vi "Trio - Set Connection Parameters.vi"(9 "TrioData In":T1 {"A Axis Parameters"."VPSPEED" format="%#_4g"; "A Axis Parameters"."AXISSTATUS" format="%#_4g"; "A Axis Parameters"."FE" format="%#_4g"; "A Axis Parameters"."MPOS" format="%#_4g"; "A Axis Parameters"."NTYPE" format="%#_4g"; "A Axis Parameters"."MTYPE" format="%#_4g"; "A Axis Parameters"."RS_LIMIT" format="%#_4g"; "A Axis Parameters"."FS_LIMIT" format="%#_4g"; "A Axis Parameters"."FH_IN" format="%#_4g"; "A Axis Parameters"."DATUM_IN" format="%#_4g"; "A Axis Parameters"."REV_IN" format="%#_4g"; "A Axis Parameters"."FWD_IN" format="%#_4g"; "A Axis Parameters"."REP_DIST" format="%#_4g"; "A Axis Parameters"."SERVO" format="%#_4g"; "A Axis Parameters"."DAC" format="%#_4g"; "A Axis Parameters"."FE_LIMIT" format="%#_4g"; "A Axis Parameters"."JOGSPEED" format="%#_4g"; "A Axis Parameters"."CREEP" format="%#_4g"; "A Axis Parameters"."DECEL" format="%#_4g"; "A Axis Parameters"."ACCEL" format="%#_4g"; "A Axis Parameters"."SPEED" format="%#_4g"; "A Axis Parameters"."UNITS" format="%#_4g"; "A Axis Parameters"."VFF_GAIN" format="%#_4g"; "A Axis Parameters"."0V_GAIN" format="%#_4g"; "A Axis Parameters"."D_GAIN" format="%#_4g"; "A Axis Parameters"."I_GAIN" format="%#_4g"; "A Axis Parameters"."P_GAIN" format="%#_4g"; "A Axis Parameters"."ATYPE" format="%#_4g"; "X Axis Parameters"."VPSPEED" format="%#_4g"; "X Axis Parameters"."AXISSTATUS" format="%#_4g"; "X Axis Parameters"."FE" format="%#_4g"; "X Axis Parameters"."MPOS" format="%#_4g"; "X Axis Parameters"."NTYPE" format="%#_4g"; "X Axis Parameters"."MTYPE" format="%#_4g"; "X Axis Parameters"."RS_LIMIT" format="%#_4g"; "X Axis Parameters"."FS_LIMIT" format="%#_4g"; "X Axis Parameters"."FH_IN" format="%#_4g"; "X Axis Parameters"."DATUM_IN" format="%#_4g"; "X Axis Parameters"."REV_IN" format="%#_4g"; "X Axis Parameters"."FWD_IN" format="%#_4g"; "X Axis Parameters"."REP_DIST" format="%#_4g"; "X Axis Parameters"."SERVO" format="%#_4g"; "X Axis Parameters"."DAC" format="%#_4g"; "X Axis Parameters"."FE_LIMIT" format="%#_4g"; "X Axis Parameters"."JOGSPEED" format="%#_4g"; "X Axis Parameters"."CREEP" format="%#_4g"; "X Axis Parameters"."DECEL" format="%#_4g"; "X Axis Parameters"."ACCEL" format="%#_4g"; "X Axis Parameters"."SPEED" format="%#_4g"; "X Axis Parameters"."UNITS" format="%#_4g"; "X Axis Parameters"."VFF_GAIN" format="%#_4g"; "X Axis Parameters"."0V_GAIN" format="%#_4g"; "X Axis Parameters"."D_GAIN" format="%#_4g"; "X Axis Parameters"."I_GAIN" format="%#_4g"; "X Axis Parameters"."P_GAIN" format="%#_4g"; "X Axis Parameters"."ATYPE" format="%#_4g"}, 10 "error in (no error)":errorcluster, 11 "TrioControl Refnum in":refnum<k7>) -> (1 "TrioData Out":T1 {"A Axis Parameters"."VPSPEED" format="%#_4g"; "A Axis Parameters"."AXISSTATUS" format="%#_4g"; "A Axis Parameters"."FE" format="%#_4g"; "A Axis Parameters"."MPOS" format="%#_4g"; "A Axis Parameters"."NTYPE" format="%#_4g"; "A Axis Parameters"."MTYPE" format="%#_4g"; "A Axis Parameters"."RS_LIMIT" format="%#_4g"; "A Axis Parameters"."FS_LIMIT" format="%#_4g"; "A Axis Parameters"."FH_IN" format="%#_4g"; "A Axis Parameters"."DATUM_IN" format="%#_4g"; "A Axis Parameters"."REV_IN" format="%#_4g"; "A Axis Parameters"."FWD_IN" format="%#_4g"; "A Axis Parameters"."REP_DIST" format="%#_4g"; "A Axis Parameters"."SERVO" format="%#_4g"; "A Axis Parameters"."DAC" format="%#_4g"; "A Axis Parameters"."FE_LIMIT" format="%#_4g"; "A Axis Parameters"."JOGSPEED" format="%#_4g"; "A Axis Parameters"."CREEP" format="%#_4g"; "A Axis Parameters"."DECEL" format="%#_4g"; "A Axis Parameters"."ACCEL" format="%#_4g"; "A Axis Parameters"."SPEED" format="%#_4g"; "A Axis Parameters"."UNITS" format="%#_4g"; "A Axis Parameters"."VFF_GAIN" format="%#_4g"; "A Axis Parameters"."0V_GAIN" format="%#_4g"; "A Axis Parameters"."D_GAIN" format="%#_4g"; "A Axis Parameters"."I_GAIN" format="%#_4g"; "A Axis Parameters"."P_GAIN" format="%#_4g"; "A Axis Parameters"."ATYPE" format="%#_4g"; "X Axis Parameters"."VPSPEED" format="%#_4g"; "X Axis Parameters"."AXISSTATUS" format="%#_4g"; "X Axis Parameters"."FE" format="%#_4g"; "X Axis Parameters"."MPOS" format="%#_4g"; "X Axis Parameters"."NTYPE" format="%#_4g"; "X Axis Parameters"."MTYPE" format="%#_4g"; "X Axis Parameters"."RS_LIMIT" format="%#_4g"; "X Axis Parameters"."FS_LIMIT" format="%#_4g"; "X Axis Parameters"."FH_IN" format="%#_4g"; "X Axis Parameters"."DATUM_IN" format="%#_4g"; "X Axis Parameters"."REV_IN" format="%#_4g"; "X Axis Parameters"."FWD_IN" format="%#_4g"; "X Axis Parameters"."REP_DIST" format="%#_4g"; "X Axis Parameters"."SERVO" format="%#_4g"; "X Axis Parameters"."DAC" format="%#_4g"; "X Axis Parameters"."FE_LIMIT" format="%#_4g"; "X Axis Parameters"."JOGSPEED" format="%#_4g"; "X Axis Parameters"."CREEP" format="%#_4g"; "X Axis Parameters"."DECEL" format="%#_4g"; "X Axis Parameters"."ACCEL" format="%#_4g"; "X Axis Parameters"."SPEED" format="%#_4g"; "X Axis Parameters"."UNITS" format="%#_4g"; "X Axis Parameters"."VFF_GAIN" format="%#_4g"; "X Axis Parameters"."0V_GAIN" format="%#_4g"; "X Axis Parameters"."D_GAIN" format="%#_4g"; "X Axis Parameters"."I_GAIN" format="%#_4g"; "X Axis Parameters"."P_GAIN" format="%#_4g"; "X Axis Parameters"."ATYPE" format="%#_4g"}, 2 "error out":errorcluster, 3 "TrioControl Refnum Out":refnum<k7>)   [LabVIEW 2020, in "TrioMotion Controller.lvlib"]
uses:
  TrioMotion Controller.lvlib
  TrioData.ctl
  Connection Type.ctl
  Axis Parameters.ctl
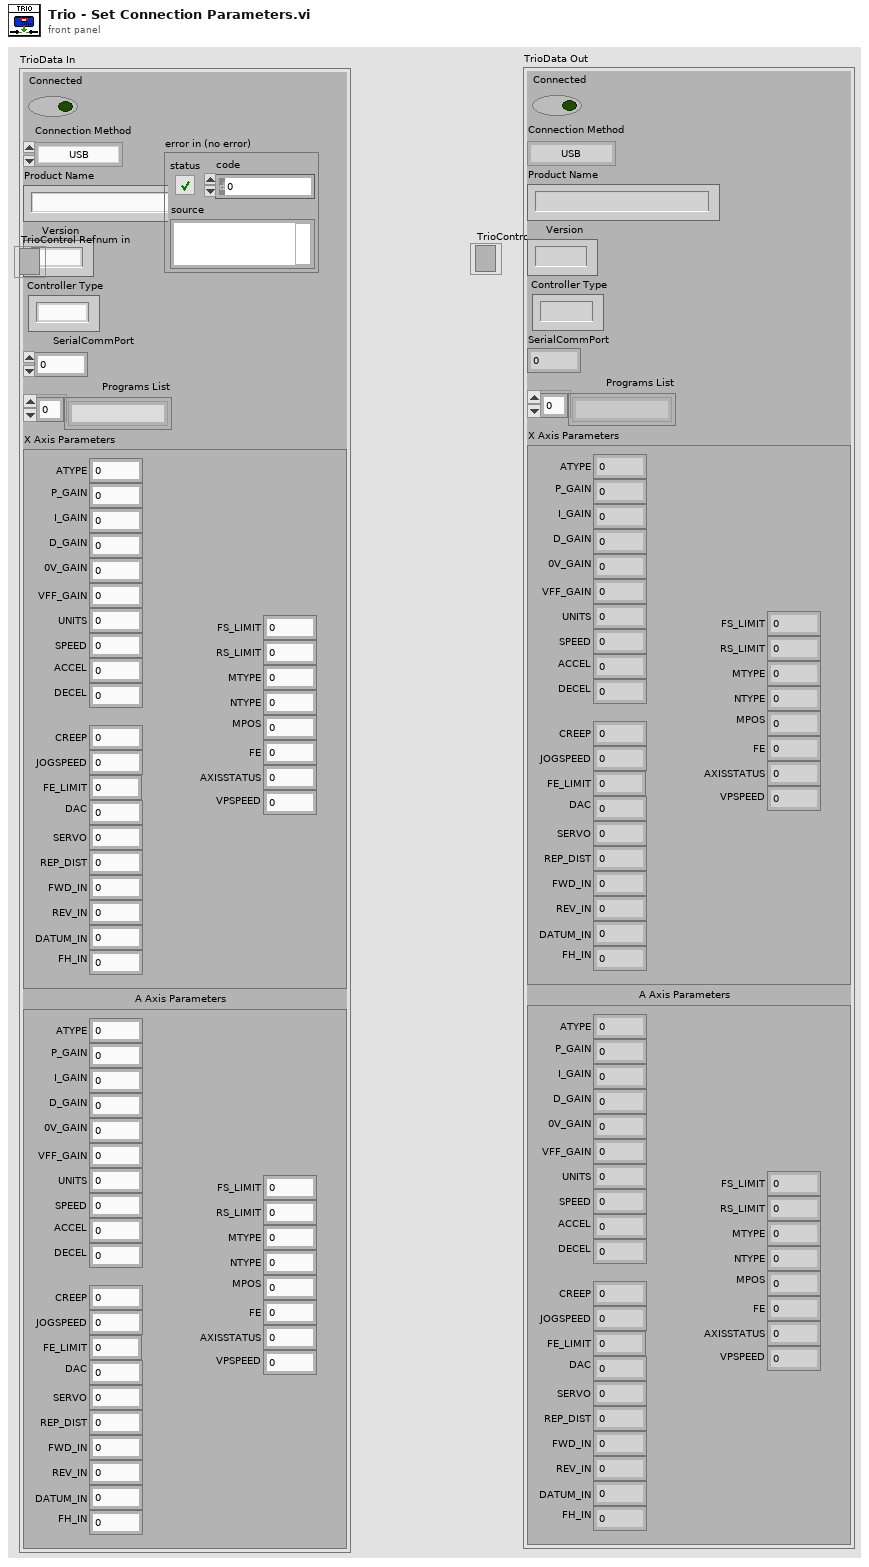
[diagram p1: front panel]
types:
  T1 = typedef "TrioMotion Controller.lvlib/TrioData.ctl" = cluster{"Connected":bool, "Connection Method":T2, "Product Name":string, " Version":string, "Controller Type":string, "SerialCommPort":fxp<+,3,3>, "Programs List":string[], "X Axis Parameters":T3, "A Axis Parameters":T3}
  T2 = typedef "TrioMotion Controller.lvlib/Connection Type.ctl" = enum16{"USB", "Serial", "Ethernet", "PCI", "Path", "No connection"}
  T3 = typedef "TrioMotion Controller.lvlib/Axis Parameters.ctl" = cluster{"ATYPE":dbl, "P_GAIN":dbl, "I_GAIN":dbl, "D_GAIN":dbl, "0V_GAIN":dbl, "VFF_GAIN":dbl, "UNITS":dbl, "SPEED":dbl, "ACCEL":dbl, "DECEL":dbl, "CREEP":dbl, "JOGSPEED":dbl, "FE_LIMIT":dbl, "DAC":dbl, "SERVO":dbl, "REP_DIST":dbl, "FWD_IN":dbl, "REV_IN":dbl, "DATUM_IN":dbl, "FH_IN":dbl, "FS_LIMIT":dbl, "RS_LIMIT":dbl, "MTYPE":dbl, "NTYPE":dbl, "MPOS":dbl, "FE":dbl, "AXISSTATUS":dbl, "VPSPEED":dbl}
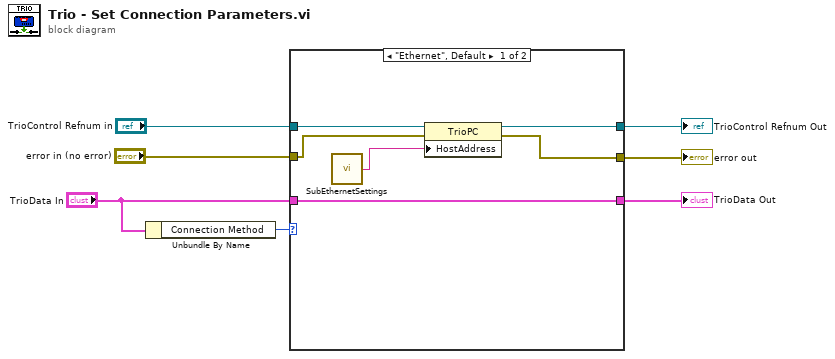
[diagram p0: block diagram]
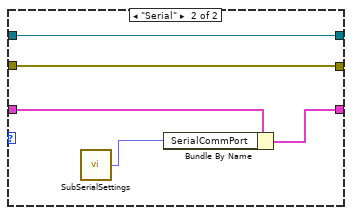
[diagram p2: hidden frame]
diagram:
  n1 = Unbundle By Name("TrioData In") -> ("Connection Method"=w7:T2)
  n2 = case shown="\"Ethernet\", Default" w7 {
    tunnel: "TrioControl Refnum in" -> [w12 w15]
    tunnel: "error in (no error)" -> [w11 w14]
    tunnel: [w10 w15] -> w4
    tunnel: [w9 w14] -> w3
    tunnel: "TrioData In" -> [w8 w17]
    tunnel: [w8 w16] -> w1
    frame "Ethernet", Default {
      n3 = call "SubEthernetSettings.vi"() -> ("Ethernet IP Address 2"=w13:string)
      n4 = property class="TrioPC"(reference=w12, error in=w11, "HostAddress"=w13) -> (reference out=w10:refnum<k7>, error out=w9:errorcluster)
    }
    frame "Serial" {
      n5 = call "SubSerialSettings.vi"() -> ("CommPort"=w18:fxp<+,3,3>)
      n6 = Bundle By Name(cluster=w17, "SerialCommPort"=w18) -> (w16:T1)
    }
  }
  "TrioControl Refnum Out" <- w4
  "error out" <- w3
  "TrioData Out" <- w1
